vi "binary_write.vi"(0 "Byte Stream File in":refnum<file>, 1 "UserData":sgl, 2 "EODText":string, 3 "Polarity":i8, 4 "prepend array or string size? (T)":bool, 5 "error in (no error)":errorcluster, 6 "Sample Rate":i32, 7 "NBytes":i8, 8 "AD Range":sgl, 9 "NBits":i8, 10 "nPts":i32, 11 "byte order (0:big-endian, network order)":T1(ring), 12 "WaveformData":i16[](array[numeric]), 13 "Version":i8) -> (14 "Byte Stream File out":refnum<file>, 19 "error out":errorcluster)   [LabVIEW 2014]
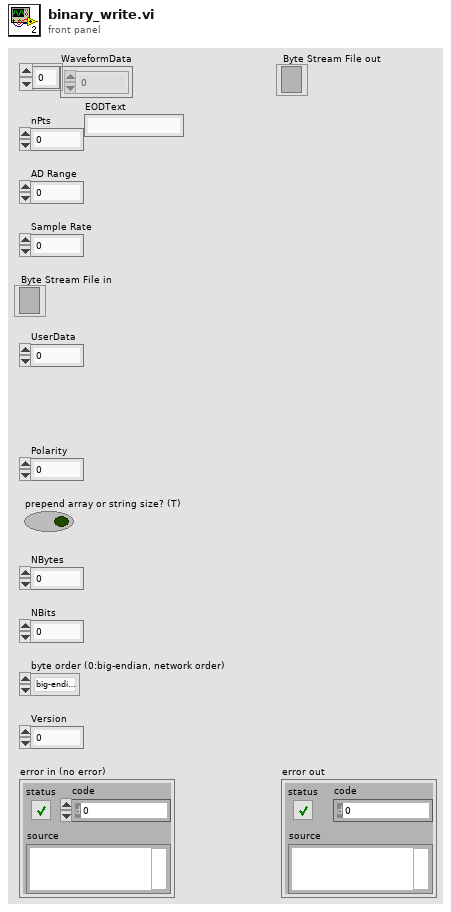
[diagram p1: front panel]
types:
  T1 = enum16{"big-endian, network order", "native, host order", "little-endian"}
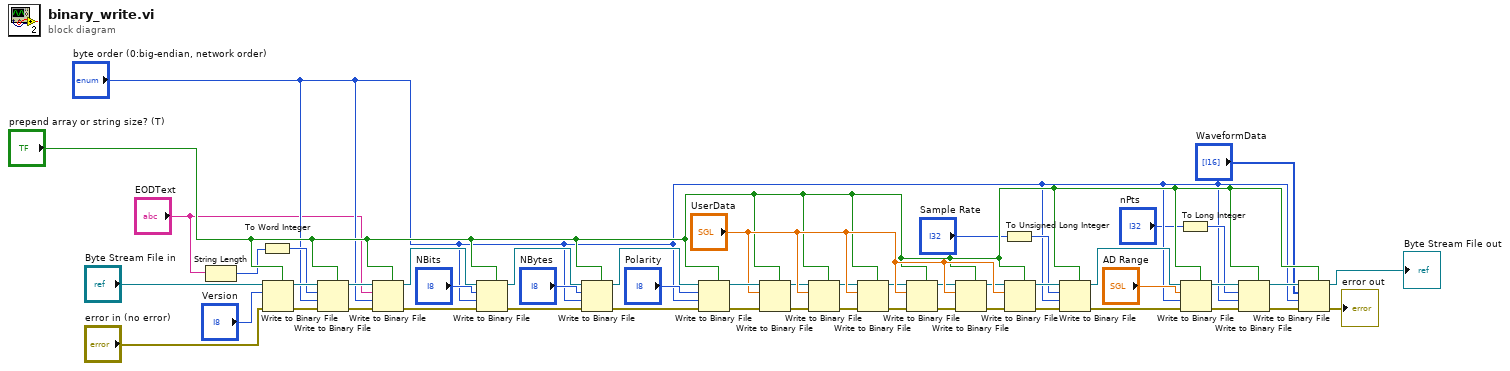
[diagram p0: block diagram]
diagram:
  n1 = String Length(string="EODText") -> (length=w2:i32)
  n2 = To Word Integer(number=w2) -> (16bit integer=w7:i16)
  n3 = Write to Binary File(file (use dialog)="Byte Stream File in", data="Version", error in="error in (no error)", 5:"prepend array or string size? (T)") -> (refnum out=w30:refnum<file>, error out=w29:errorcluster)  [unwired: 2 in, 1 out]
  n4 = Write to Binary File(file (use dialog)=w30, data=w7, error in=w29, 5:"prepend array or string size? (T)", 9:"byte order (0:big-endian, network order)") -> (refnum out=w17:refnum<file>, error out=w18:errorcluster)  [unwired: 1 in, 1 out]
  n5 = Write to Binary File(file (use dialog)=w17, data="EODText", error in=w18, 5:"prepend array or string size? (T)", 9:"byte order (0:big-endian, network order)") -> (refnum out=w31:refnum<file>, error out=w32:errorcluster)  [unwired: 1 in, 1 out]
  n6 = Write to Binary File(file (use dialog)=w31, data="NBits", error in=w32, 5:"prepend array or string size? (T)", 9:"byte order (0:big-endian, network order)") -> (refnum out=w27:refnum<file>, error out=w19:errorcluster)  [unwired: 1 in, 1 out]
  n7 = Write to Binary File(file (use dialog)=w27, data="NBytes", error in=w19, 5:"prepend array or string size? (T)", 9:"byte order (0:big-endian, network order)") -> (refnum out=w28:refnum<file>, error out=w20:errorcluster)  [unwired: 1 in, 1 out]
  n8 = Write to Binary File(file (use dialog)=w28, data="Polarity", error in=w20, 5:"prepend array or string size? (T)", 9:"byte order (0:big-endian, network order)") -> (refnum out=w47:refnum<file>, error out=w48:errorcluster)  [unwired: 1 in, 1 out]
  n9 = Write to Binary File(file (use dialog)=w47, data="UserData", error in=w48, 5:"prepend array or string size? (T)") -> (refnum out=w40:refnum<file>, error out=w35:errorcluster)  [unwired: 2 in, 1 out]
  n10 = Write to Binary File(file (use dialog)=w40, data="UserData", error in=w35, 5:"prepend array or string size? (T)") -> (refnum out=w41:refnum<file>, error out=w36:errorcluster)  [unwired: 2 in, 1 out]
  n11 = Write to Binary File(file (use dialog)=w41, data="UserData", error in=w36, 5:"prepend array or string size? (T)") -> (refnum out=w42:refnum<file>, error out=w37:errorcluster)  [unwired: 2 in, 1 out]
  n12 = Write to Binary File(file (use dialog)=w42, data="UserData", error in=w37, 5:"prepend array or string size? (T)") -> (refnum out=w43:refnum<file>, error out=w38:errorcluster)  [unwired: 2 in, 1 out]
  n13 = Write to Binary File(file (use dialog)=w43, data="UserData", error in=w38, 5:"prepend array or string size? (T)") -> (refnum out=w44:refnum<file>, error out=w39:errorcluster)  [unwired: 2 in, 1 out]
  n14 = To Unsigned Long Integer(number="Sample Rate") -> (unsigned 32bit integer=w10:u32)
  n15 = Write to Binary File(file (use dialog)=w44, data="UserData", error in=w39, 5:"prepend array or string size? (T)") -> (refnum out=w49:refnum<file>, error out=w50:errorcluster)  [unwired: 2 in, 1 out]
  n16 = Write to Binary File(file (use dialog)=w49, data=w10, error in=w50, 5:"prepend array or string size? (T)", 9:"byte order (0:big-endian, network order)") -> (refnum out=w21:refnum<file>, error out=w22:errorcluster)  [unwired: 1 in, 1 out]
  n17 = To Long Integer(number="nPts") -> (32bit integer=w12:i32)
  n18 = Write to Binary File(file (use dialog)=w21, data="AD Range", error in=w22, 5:"prepend array or string size? (T)", 9:"byte order (0:big-endian, network order)") -> (refnum out=w23:refnum<file>, error out=w24:errorcluster)  [unwired: 1 in, 1 out]
  n19 = Write to Binary File(file (use dialog)=w23, data=w12, error in=w24, 5:"prepend array or string size? (T)", 9:"byte order (0:big-endian, network order)") -> (refnum out=w25:refnum<file>, error out=w26:errorcluster)  [unwired: 1 in, 1 out]
  n20 = Write to Binary File(file (use dialog)=w25, data="WaveformData", error in=w26, 5:"prepend array or string size? (T)", 9:"byte order (0:big-endian, network order)") -> (refnum out=→"Byte Stream File out":refnum<file>, error out=→"error out":errorcluster)  [unwired: 1 in, 1 out]
